vi "Set_up_process_notifiers.vi"(11 "Process notifier names":string[](array[string])=["drive", "gear", "elevator"]) -> (3 "Notifier Refnums":refnum<notifier>[](array[refnum]), 4 "All done array":string[](array[string]))   [LabVIEW 2017, in "labview-standard-library.lvlib" / "automode-scripting.lvlib"]
uses:
  automode-scripting.lvlib
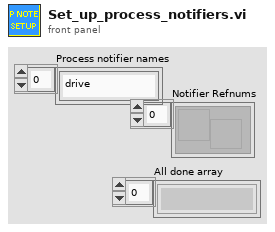
[diagram p1: front panel]
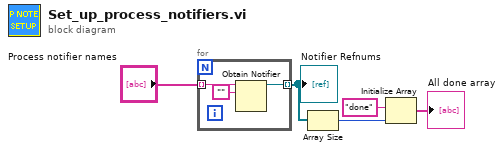
[diagram p0: block diagram]
diagram:
  n1 = for {
    tunnel: "Process notifier names" -> [w7] mode=indexing
    tunnel: [w6] -> w1 mode=indexing
    n2 = Obtain Notifier(name (unnamed)=w7, notification data type="") -> (notifier out=w6:refnum<notifier>)  [unwired: 2 in, 2 out]
  }
  "Notifier Refnums" <- w1
  n3 = Array Size(array=w1) -> (size(s)=w2:i32)
  n4 = Initialize Array("done", w2) -> (→"All done array":string[])
